vi "image labeler interface.vi"() -> ()   [LabVIEW 2009]
panel:
  out "Progress":i32(slide) scale=0.0..10.0
  out "new picture":picture
  in  "text":string
  in  "[user-specified font]":T1={"Font Name:"="helvetica", "Size"=18, "Strikeout?"=FALSE, "Italic?"=FALSE, "Underline?"=FALSE, "Outline?"=FALSE, "Shadow?"=FALSE, "Bold?"=FALSE}
  in  "image types":cluster{".png":bool, ".jpeg":bool, ".bmp":bool}={".png"=TRUE, ".jpeg"=TRUE, ".bmp"=TRUE}
  in  "path":path
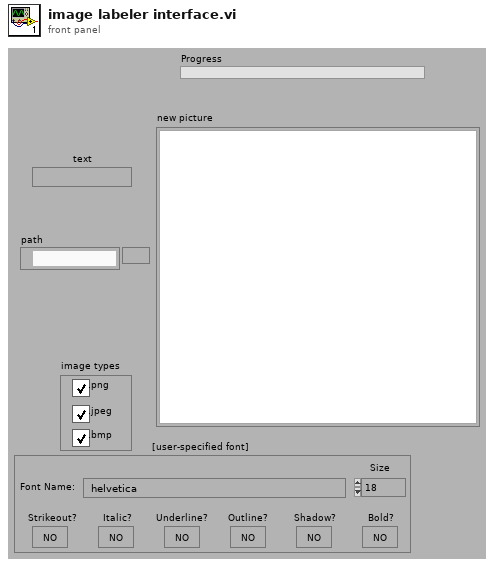
[diagram p1: front panel]
types:
  T1 = cluster{"Font Name:":string, "Size":i16, "Strikeout?":bool, "Italic?":bool, "Underline?":bool, "Outline?":bool, "Shadow?":bool, "Bold?":bool}
  T2 = typedef "imagedata.ctl" = cluster{"image type":i32, "image depth":i32, "image":u8[], "mask":u8[], "colors":u32[], "Rectangle":cluster{"left":i16, "top":i16, "right":i16, "bottom":i16}}
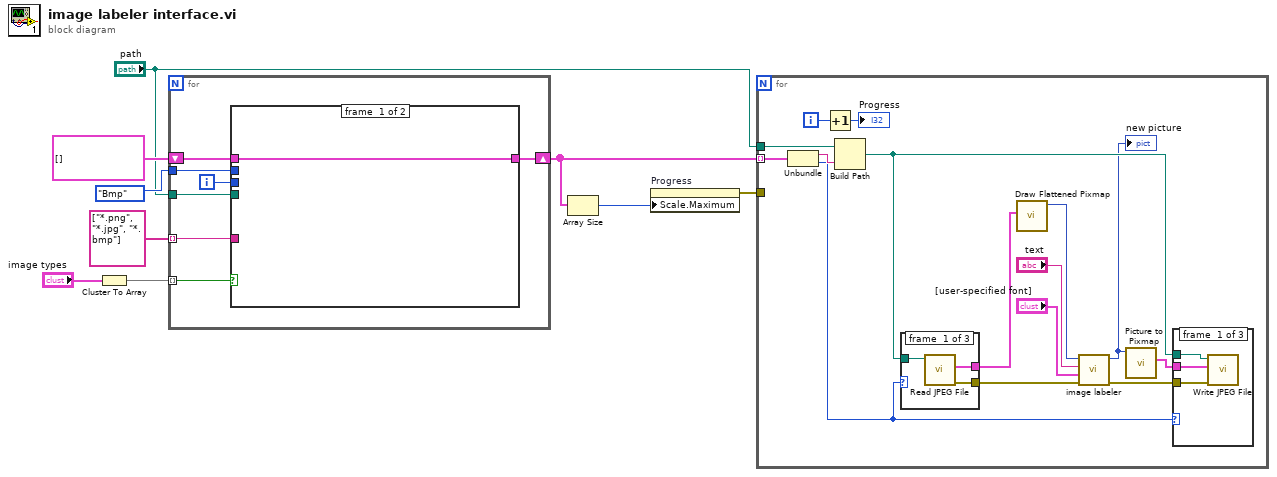
[diagram p0: block diagram]
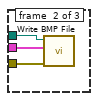
[diagram p2: hidden frame]
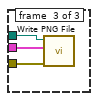
[diagram p3: hidden frame]
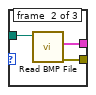
[diagram p4: hidden frame]
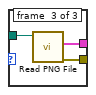
[diagram p5: hidden frame]
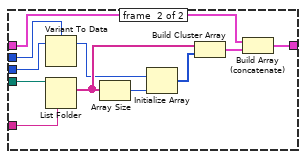
[diagram p6: hidden frame]
diagram:
  n1 = Cluster To Array(cluster="image types") -> (array=w7:bool[])
  n2 = for {
    tunnel: string[] ["*.png", "*.jpg", "*.bmp"] ("appended array") -> [w15] mode=indexing
    tunnel: w7 -> [w10] mode=indexing
    tunnel: "path" -> [w16]
    tunnel: enum8{"PNG", "Jpeg", "Bmp"}."Bmp" -> [w14]
    shift-right: [w12] -> w3
    shift-left: cluster{string, enum8{"PNG", "Jpeg", "Bmp"}}[] [] -> [w11]
    i -> [w13]
    n3 = case shown="True" w10 {
      tunnel: w16 -> [_ w28]
      tunnel: w15 -> [_ w27]
      tunnel: w14 -> [_ w26]
      tunnel: w13 -> [_ w25]
      tunnel: [w17 w19] -> w12
      tunnel: w11 -> [w17 w18]
      frame #0 {
      }
      frame #1 {
        n4 = Variant To Data(Variant=w25, type=w26) -> (data=w23:enum8{"PNG", "Jpeg", "Bmp"})  [unwired: 1 in, 1 out]
        n5 = List Folder(path=w28, pattern=w27) -> (filenames=w24:string[])  [unwired: 2 in, 3 out]
        n6 = Array Size(array=w24) -> (size(s)=w22:i32)
        n7 = Initialize Array(w23, w22) -> (w21:enum8{"PNG", "Jpeg", "Bmp"}[])
        n8 = Build Cluster Array(w24, w21) -> (w20:cluster{string, enum8{"PNG", "Jpeg", "Bmp"}}[])
        n9 = Build Array (concatenate)(w18, w20) -> (w19:cluster{string, enum8{"PNG", "Jpeg", "Bmp"}}[])
      }
    }
  }
  n10 = Array Size(array=w3) -> (size(s)=w1:i32)
  n11 = property on="Progress" class="Slide (strict)"("Scale.Maximum"=w1) -> (error out=w2:errorcluster)  [unwired: 2 in, 1 out]
  n12 = for {
    tunnel: w3 -> [w38] mode=indexing
    tunnel: "path" -> [w36]
    tunnel: w2 -> [_]
    i -> [w30]
    n13 = Unbundle(w38) -> (w37:string, w35:enum8{"PNG", "Jpeg", "Bmp"})
    n14 = Increment(x=w30) -> (x+1=→"Progress":i32)
    n15 = Build Path(base path=w36, name or relative path=w37) -> (appended path=w34:path)
    n16 = case shown="\"PNG\"" w35 {
      tunnel: [w55 w58 w61] -> w41
      tunnel: [w54 w57 w60] -> w39
      tunnel: w34 -> [w53 w56 w59]
      frame #0 {
        n17 = call <vilib>:"Read JPEG File.vi"("path to JPEG file"=w53) -> ("error out"=w54:errorcluster, "image data"=w55:T2)  [unwired: 8 in, 1 out]
      }
      frame #1 {
        n18 = call <vilib>:"Read BMP File.vi"("path to BMP file"=w56) -> ("error out"=w57:errorcluster, "image data"=w58:T2)  [unwired: 8 in, 1 out]
      }
      frame #2 {
        n19 = call <vilib>:"Read PNG File.vi"("path to PNG file"=w59) -> ("error out"=w60:errorcluster, "image data"=w61:T2)  [unwired: 8 in, 1 out]
      }
    }
    n20 = call <vilib>:"Draw Flattened Pixmap.vi"("image data"=w41) -> ("new picture"=w40:picture)  [unwired: 8 in]
    n21 = call "image labeler.vi"("error in (no error)"=w39, "[user-specified font]"="[user-specified font]", "text"="text", "picture"=w40) -> ("error out"=w31:errorcluster, "new picture"=w32:picture)  [unwired: 6 in]
    "new picture" <- w32
    n22 = call <vilib>:"Picture to Pixmap.vi"("picture"=w32) -> ("image data"=w33:T2)  [unwired: 9 in, 1 out]
    n23 = case shown="\"Jpeg\"" w35 {
      tunnel: w34 -> [w46 w49 w52]
      tunnel: w33 -> [w45 w48 w51]
      tunnel: w31 -> [w44 w47 w50]
      frame #0 {
        n24 = call <vilib>:"Write JPEG File.vi"("error in (no error)"=w44, "image data"=w45, "path to JPEG file"=w46) -> ()  [unwired: 7 in, 2 out]
      }
      frame #1 {
        n25 = call <vilib>:"Write BMP File.vi"("error in (no error)"=w47, "image data"=w48, "path to BMP file"=w49) -> ()  [unwired: 7 in, 2 out]
      }
      frame #2 {
        n26 = call <vilib>:"Write PNG File.vi"("error in (no error)"=w50, "image data"=w51, "path to PNG file"=w52) -> ()  [unwired: 7 in, 2 out]
      }
    }
  }
